vi "5.8G_Range Profile_audiojack_FMCW_demo_exe.vi"() -> ()   [LabVIEW 2015]
doc: "This example demonstrates how to use the Short-time Fourier Transform (STFT Spectrograms) VI to analyze the Time-Frequency spectrogram."
uses:
  <vilib>/Analysis/baseanly.llb/Unit Vector (DBL).vi
  <vilib>/Analysis/baseanly.llb/Mean (DBL).vi
  <vilib>/Analysis/2dsp.llb/Real FFT.vi
  <vilib>/Analysis/2dsp.llb/Complex FFT.vi
  <vilib>/Analysis/0measdsp.llb/Scaled Time Domain Window (DBL).vi
  <vilib>/sound2/lvsound2.llb/Sound Input Read (DBL).vi
  <vilib>/Analysis/NI_AALPro.lvlib
  <vilib>/Analysis/NI_AALBase.lvlib
panel:
  in  "begin offsets":i32=10
  in  "end offsets":i32=200
  in  "window":u32(ring)=1 items=["Rectangle"=0, "Hanning"=1, "Hamming"=2, "Blackman-Harris"=3, "Exact Blackman"=4, "Blackman"=5, "Flat Top"=6, "4 Term B-Harris "=7, "7 Term B-Harris"=8, "Low Sidelobe"=9, "Blackman Nuttall"=11, "Triangle"=30, "Bartlett-Hanning"=31, "Bohman"=32, "Parzen"=33, "Welch"=34, "Kaiser"=60, "Dolph-Chebyshev"=61, "Gaussian"=62]
  in  "ISAR intensify:Minimum":dbl=-30.0
  in  "ISAR intensify: Maximum":dbl
  in  "map selector ISAR":T1(ring)=enum."rainbow"
  out "ISAR":dbl[][](graph)
  in  "range":dbl(slide)=8.722182340272793 min=0.0 max=128.57142857142858 scale=0.0..128.57142857142858
  out "max range":dbl
  out "range resolution":dbl
  out "chirp rate":dbl
  in  "Range intensify:Minimum":dbl=-40.0
  in  "Range intensify:Maximum":dbl
  out "real time chirp frequency":dbl
  in  "FFT length":i32=4096
  in  "chirp frequency":dbl=280.0
  out "Range profile":dbl[][](graph)
  out "average samples per chirp":i32
  in  "threshold":dbl=0.6 format="%0.2f"
  in  "bits per sample":i32=16
  in  "number of channels":i32=2
  in  "sample rate (S/s)":dbl=192000.0
  in  "data length\n(10 x number of samples/ch)":i32=400000 min=10000 max=1000000
  in  "map selector Range profile":T1(ring)=enum."rainbow"
  in  "number of samples/ch":i32=40000 min=1024 max=100000
  in  "Numeric Control":dbl=1.0
  in  "device ID":u32
  in  "Stop":bool
  # "FMCW Radar Realtime Range Detection and ISAR Video"
  # "Version: 4\nZhengyu Peng\nC. Li Lab\nTexas Tech University\nOct. 2016"
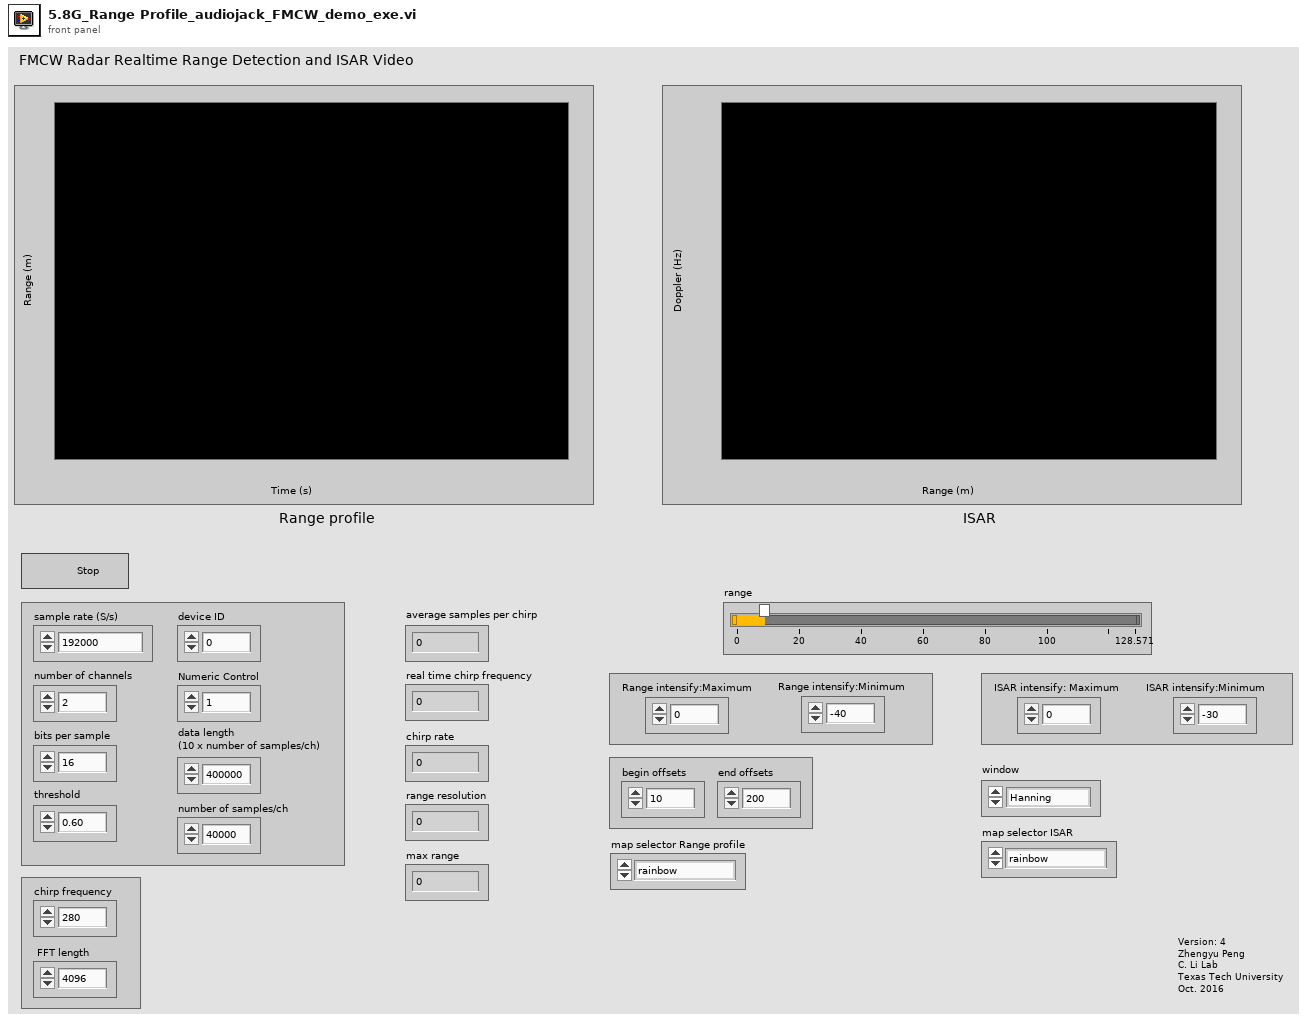
[diagram p1: front panel]
types:
  T1 = enum16{"fire", "rainbow", "grey", "inverse grey", "ice", "original"}
  T2 = cluster{"sample rate (S/s)":dbl, "number of channels":i32, "bits per sample ":i32}
  T3 = typedef "Sound Input Task ID.ctl" = u32
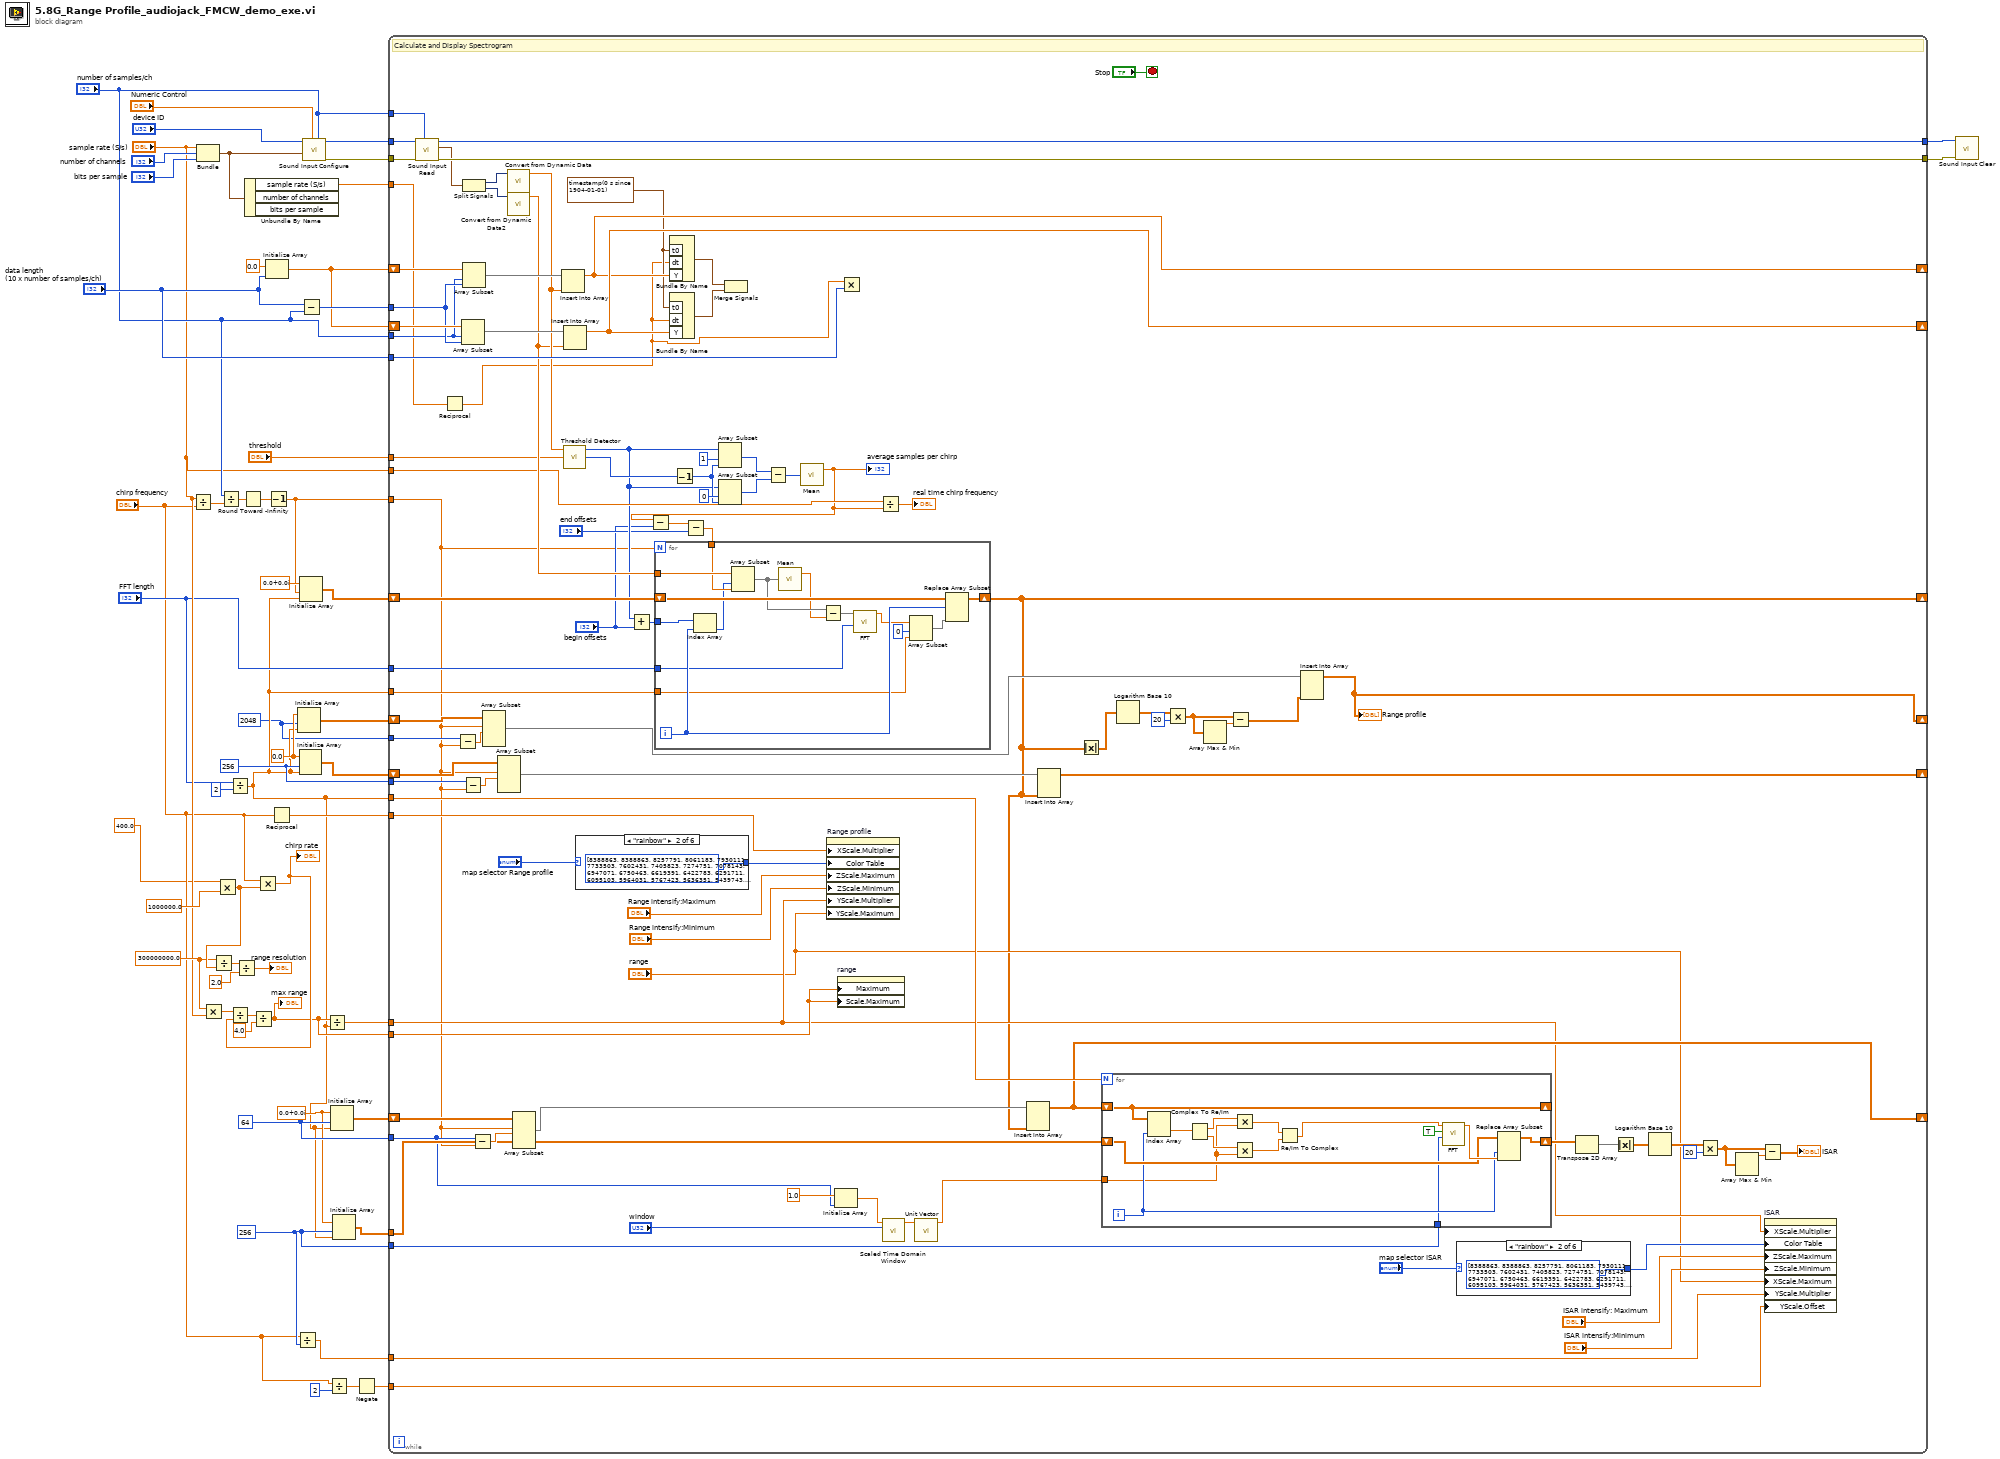
[diagram p0: block diagram]
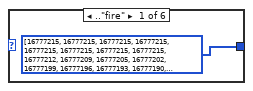
[diagram p2: hidden frame]
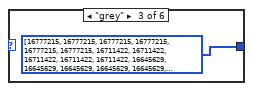
[diagram p3: hidden frame]
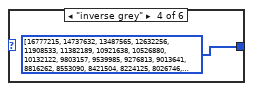
[diagram p4: hidden frame]
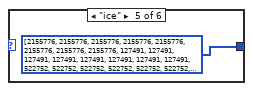
[diagram p5: hidden frame]
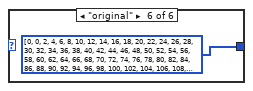
[diagram p6: hidden frame]
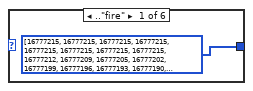
[diagram p7: hidden frame]
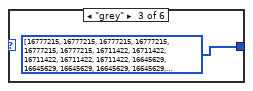
[diagram p8: hidden frame]
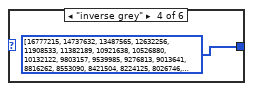
[diagram p9: hidden frame]
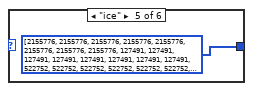
[diagram p10: hidden frame]
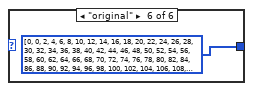
[diagram p11: hidden frame]
diagram:
  w1 = 2048 ("dimension size")
  w7 = 256 ("dimension size")
  w14 = 64 ("dimension size")
  w13 = cdb 0.0+0.0i ("element")
  w25 = 300000000.0 ("x")
  w32 = 256 ("dimension size")
  w4 = 0.0 ("element")
  n1 = Divide(x="sample rate (S/s)", y="chirp frequency") -> (x/y=w36:dbl)
  n2 = Bundle("sample rate (S/s)"="sample rate (S/s)", "number of channels"="number of channels", "bits per sample"="bits per sample") -> (w43:T2)  [unwired: 1 in]
  n3 = Multiply(x=w25, y="sample rate (S/s)") -> (x*y=w24:dbl)
  n4 = Multiply(x=400.0, y=1000000.0) -> (x*y=w29:dbl)
  n5 = Divide(x=w25, y=w29) -> (x/y=w28:dbl)
  n6 = Divide(x="number of samples/ch", y=w36) -> (x/y=w35:dbl)
  n7 = Divide(x="FFT length", y=2) -> (x/y=w3:dbl)
  n8 = Divide(x=w28, y=2.0) -> (x/y=→"range resolution":dbl)
  n9 = Round Toward -Infinity(1:w35) -> (0:w34:dbl)
  n10 = Unbundle By Name(w43) -> ("sample rate (S/s)"=w46:dbl)  [unwired: 2 out]
  n11 = Multiply(x="chirp frequency", y=w29) -> (x*y=w23:dbl)
  "chirp rate" <- w23
  n12 = Divide(x=w24, y=w23) -> (x/y=w22:dbl)
  n13 = Divide(x=w22, y=4.0) -> (x/y=w16:dbl)
  "max range" <- w16
  n14 = Initialize Array(0.0 ("element"), "data length\n(10 x number of samples/ch)") -> (w47:dbl[])
  n15 = Decrement(x=w34) -> (x-1=w33:dbl)
  n16 = Reciprocal(x="chirp frequency") -> (1/x=w31:dbl)
  n17 = Divide(x="chirp frequency", y=w7) -> (x/y=w8:dbl)
  n18 = Initialize Array(w4, w1, w3) -> (w2:dbl[][])
  n19 = Initialize Array(w4, w32, w3) -> (w41:dbl[][])
  n20 = Subtract(x="data length\n(10 x number of samples/ch)", y="number of samples/ch") -> (x-y=w48:i32)
  n21 = Initialize Array(cdb 0.0+0.0i ("element"), w33, w3) -> (w39:cdb[][])
  n22 = call <vilib>:"Sound Input Configure.vi"("number of samples/ch"="number of samples/ch", "sample mode"="Numeric Control", "sound format"=w43, "device ID"="device ID") -> ("error out"=w52:errorcluster, "task ID"=w54:T3)  [unwired: 6 in]
  n23 = Divide(x=w16, y=w3) -> (x/y=w17:dbl)
  n24 = Divide(x="chirp frequency", y=2) -> (x/y=w10:dbl)
  n25 = Initialize Array(w13, w14, w3) -> (w15:cdb[][])
  n26 = Initialize Array(w13, w7, w3) -> (w12:cdb[][])
  n27 = Negate(x=w10) -> (-x=w9:dbl)
  n28 = while {
    tunnel: w54 -> [w152]
    tunnel: "number of samples/ch" -> [w151]
    tunnel: w52 -> [w150]
    tunnel: [w149] -> w51
    tunnel: [w148] -> w50
    shift-right: [w132] -> _
    shift-left: w47 -> [w144]
    tunnel: w48 -> [w141]
    shift-right: [w134] -> _
    shift-left: w47 -> [w142]
    tunnel: "number of samples/ch" -> [w137]
    tunnel: w46 -> [w133]
    tunnel: "data length\n(10 x number of samples/ch)" -> [w135]
    shift-right: [w60] -> _
    shift-left: w41 -> [w123]
    shift-right: [w57] -> _
    shift-left: w39 -> [w122]
    tunnel: "threshold" -> [w113]
    tunnel: w33 -> [w62]
    tunnel: "sample rate (S/s)" -> [w112]
    tunnel: "FFT length" -> [w110]
    tunnel: w32 -> [w109]
    tunnel: w31 -> [w66]
    tunnel: w17 -> [w83]
    tunnel: w3 -> [w104]
    tunnel: w16 -> [w103]
    shift-right: [w98] -> _
    shift-left: w15 -> [w102]
    tunnel: w14 -> [w86]
    tunnel: w3 -> [w99]
    tunnel: w12 -> [w97]
    tunnel: w7 -> [w76]
    tunnel: w9 -> [w74]
    tunnel: w8 -> [w75]
    shift-right: [w56] -> _
    shift-left: w2 -> [w65]
    tunnel: w1 -> [w64]
    stop <- "Stop" stop-if-true
    w120 = timestamp(0 s since 1904-01-01) ("t0")
    # "Calculate and Display Spectrogram"
    n29 = call-poly <vilib>:"Sound Input Read.vi"("number of samples/ch"=w151, "error in (no error)"=w150, "task ID"=w152) -> ("error out"=w148:errorcluster, "data"=w145:waveform(dbl)[], "task ID out"=w149:T3)  [unwired: 6 in]
    n30 = Reciprocal(x=w133) -> (1/x=w119:dbl)
    n31 = Subtract(x=w64, y=w62) -> (x-y=w63:dbl)
    n32 = Array Subset(array=w142, index=w137, length=w141) -> (w140:dbl[])
    n33 = Subtract(x=w109, y=w62) -> (x-y=w108:dbl)
    n34 = Split Signals(w145) -> (w147:dynamicdata, w146:dynamicdata)  [unwired: 2 out]
    n35 = Array Subset(array=w144, index=w137, length=w141) -> (w143:dbl[])
    n36 = Subtract(x=w86, y=w62) -> (x-y=w101:dbl)
    n37 = Array Subset(array=w65, index (row)=w62, length (row)=w63) -> (w59:dbl[][])  [unwired: 2 in]
    n38 = Array Subset(array=w123, index (row)=w62, length (row)=w108) -> (w118:dbl[][])  [unwired: 2 in]
    n39 = call "Convert from Dynamic Data"("Dynamic Data Type"=w147) -> ("Array"=w131:dbl[])  [unwired: 3 out]
    n40 = call "Convert from Dynamic Data2"("Dynamic Data Type"=w146) -> ("Array"=w121:dbl[])  [unwired: 3 out]
    n41 = Array Subset(array=w102, index (row)=w62, length (row)=w101) -> (w100:cdb[][])  [unwired: 2 in]
    n42 = Insert Into Array(array=w143, new element=w131) -> (w132:dbl[])  [unwired: 1 in]
    n43 = call <vilib>:"Threshold Detector.vi"("threshold"=w113, "X"=w131) -> ("count"=w126:i32, "Indices"=w73:i32[])  [unwired: 1 in, 1 out]
    n44 = Insert Into Array(array=w140, new element=w121) -> (w134:dbl[])  [unwired: 1 in]
    n45 = case shown="\"rainbow\"" "map selector Range profile" {
      tunnel: [u32[] [16777215, 16777215, 16777215, 16777215, 16777215, 16777215, 16777215, 16777215, 16777212, 16777209, 16777205, 16777202, 16777199, 16777196, 16777193, 16777190, 16777186, 16777183, 16777180, 16777177, 16777174, 16777170, 16777167, 16777164, 16777161, 16777158, 16777154, 16777151, 16777148, 16777145, 16777142, 16777139, 16777135, 16777132, 16777129, 16777126, 16777123, 16777119, 16777116, 16777113, 16777110, 16777107, 16777103, 16777100, 16777097, 16777094, 16777091, 16777088, 16777084, 16777081, 16777078, 16777075, 16777072, 16777068, 16777065, 16777062, 16777059, 16777056, 16777052, 16777049, 16777046, 16777043, 16777040, 16777037, 16777033, 16777030, 16777027, 16777024, 16777021, 16777017, 16777014, 16777011, 16777008, 16777005, 16777001, 16776998, 16776995, 16776992, 16776989, 16776986, 16776982, 16776979, 16776976, 16776973, 16776970, 16776966, 16776963, 16776960, 16776192, 16775424, 16774400, 16773632, 16772864, 16772096, 16771328, 16770560, 16769536, 16768768, 16768000, 16767232, 16766464, 16765440, 16764672, 16763904, 16763136, 16762368, 16761344, 16760576, 16759808, 16759040, 16758272, 16757504, 16756480, 16755712, 16754944, 16754176, 16753408, 16752384, 16751616, 16750848, 16750080, 16749312, 16748288, 16747520, 16746752, 16745984, 16745216, 16744448, 16743424, 16742656, 16741888, 16741120, 16740352, 16739328, 16738560, 16737792, 16737024, 16736256, 16735232, 16734464, 16733696, 16732928, 16732160, 16731392, 16730368, 16729600, 16728832, 16728064, 16727296, 16726272, 16725504, 16724736, 16723968, 16723200, 16722176, 16721408, 16720640, 16719872, 16719104, 16718336, 16717312, 16716544, 16715776, 16715008, 16714240, 16713216, 16712448, 16711680, 16515072, 16318464, 16056320, 15859712, 15663104, 15466496, 15269888, 15073280, 14811136, 14614528, 14417920, 14221312, 14024704, 13762560, 13565952, 13369344, 13172736, 12976128, 12713984, 12517376, 12320768, 12124160, 11927552, 11730944, 11468800, 11272192, 11075584, 10878976, 10682368, 10420224, 10223616, 10027008, 9830400, 9633792, 9371648, 9175040, 8978432, 8781824, 8585216, 8388608, 8126464, 7929856, 7733248, 7536640, 7340032, 7077888, 6881280, 6684672, 6488064, 6291456, 6029312, 5832704, 5636096, 5439488, 5242880, 5046272, 4784128, 4587520, 4390912, 4194304, 3997696, 3735552, 3538944, 3342336, 3145728, 2949120, 2686976, 2490368, 2293760, 2097152, 1900544, 1703936, 1441792, 1245184, 1048576, 851968, 655360, 393216, 196608, 65793, 65793, 65793, 65793, 65793, 65793, 65793, 65793, 0] ("256 fire") u32[] [8388863, 8388863, 8257791, 8061183, 7930111, 7733503, 7602431, 7405823, 7274751, 7078143, 6947071, 6750463, 6619391, 6422783, 6291711, 6095103, 5964031, 5767423, 5636351, 5439743, 5308671, 5112063, 4980991, 4784383, 4653311, 4456703, 4325631, 4129023, 3932415, 3801343, 3604735, 3473663, 3277055, 3145983, 2949375, 2818303, 2621695, 2490623, 2294015, 2162943, 1966335, 1835263, 1638655, 1507583, 1310975, 1179903, 983295, 852223, 655615, 524543, 327935, 196863, 511, 1791, 3071, 4351, 5631, 6911, 8191, 9471, 10751, 12031, 13311, 14591, 15871, 17151, 18431, 19711, 20991, 22271, 23551, 24831, 26111, 27391, 28671, 29951, 31231, 32511, 33791, 35071, 36351, 37631, 38911, 40191, 41471, 42751, 44031, 45311, 46591, 47871, 49151, 50431, 51711, 52991, 54271, 55551, 56831, 58111, 59391, 60671, 61951, 63231, 64511, 65532, 65527, 65522, 65517, 65512, 65507, 65502, 65497, 65492, 65487, 65482, 65477, 65472, 65467, 65462, 65457, 65452, 65447, 65442, 65437, 65432, 65427, 65422, 65417, 65412, 65407, 65402, 65397, 65392, 65387, 65382, 65377, 65372, 65367, 65362, 65357, 65352, 65347, 65342, 65337, 65332, 65327, 65322, 65317, 65312, 65307, 65302, 65297, 65292, 65287, 65282, 261888, 589568, 917248, 1244928, 1572608, 1900288, 2227968, 2555648, 2883328, 3211008, 3538688, 3866368, 4194048, 4521728, 4849408, 5177088, 5504768, 5832448, 6160128, 6487808, 6815488, 7143168, 7470848, 7798528, 8126208, 8453888, 8781568, 9109248, 9436928, 9764608, 10092288, 10419968, 10747648, 11075328, 11403008, 11730688, 12058368, 12386048, 12713728, 13041408, 13369088, 13696768, 14024448, 14352128, 14679808, 15007488, 15335168, 15662848, 15990528, 16318208, 16645888, 16775936, 16774656, 16773376, 16772096, 16770816, 16769536, 16768256, 16766976, 16765696, 16764416, 16763136, 16761856, 16760576, 16759296, 16758016, 16756736, 16755456, 16754176, 16752896, 16751616, 16750336, 16749056, 16747776, 16746496, 16745216, 16743936, 16742656, 16741376, 16740096, 16738816, 16737536, 16736256, 16734976, 16733696, 16732416, 16731136, 16729856, 16728576, 16727296, 16726016, 16724736, 16723456, 16722176, 16720896, 16719616, 16718336, 16717056, 16715776, 16714496, 16713216, 16711680] ("rainbow") u32[] [16777215, 16777215, 16777215, 16777215, 16777215, 16777215, 16711422, 16711422, 16711422, 16711422, 16711422, 16645629, 16645629, 16645629, 16645629, 16645629, 16645629, 16579836, 16579836, 16579836, 16579836, 16579836, 16514043, 16514043, 16514043, 16514043, 16514043, 16448250, 16448250, 16448250, 16448250, 16448250, 16316664, 16382457, 16382457, 16382457, 16382457, 16316664, 16316664, 16316664, 16316664, 16250871, 16250871, 16250871, 16250871, 16250871, 16185078, 16185078, 16185078, 16185078, 16119285, 16119285, 16119285, 16119285, 16119285, 16053492, 16053492, 16053492, 16053492, 15987699, 15987699, 15987699, 15987699, 15921906, 15987699, 15921906, 15921906, 15856113, 15856113, 15856113, 15856113, 15856113, 15790320, 15790320, 15790320, 15724527, 15724527, 15724527, 15724527, 15658734, 15658734, 15658734, 15658734, 15592941, 15592941, 15592941, 15592941, 15527148, 15527148, 15527148, 15461355, 15461355, 15461355, 15461355, 15395562, 15395562, 15395562, 15395562, 15329769, 15329769, 15329769, 15263976, 15263976, 15263976, 15198183, 15198183, 15198183, 15198183, 15132390, 15132390, 15132390, 15066597, 15066597, 15066597, 15000804, 15000804, 15000804, 14935011, 14935011, 14935011, 14869218, 14869218, 14869218, 14803425, 14803425, 14803425, 14737632, 14737632, 14671839, 14671839, 14671839, 14606046, 14606046, 14606046, 14540253, 14540253, 14540253, 14474460, 14474460, 14408667, 14408667, 14408667, 14342874, 14342874, 14277081, 14277081, 14277081, 14211288, 14211288, 14145495, 14145495, 14079702, 14079702, 14013909, 14013909, 14013909, 13948116, 13948116, 13882323, 13882323, 13816530, 13816530, 13750737, 13750737, 13684944, 13684944, 13619151, 13619151, 13553358, 13553358, 13487565, 13487565, 13421772, 13421772, 13355979, 13290186, 13290186, 13224393, 13224393, 13158600, 13092807, 13092807, 13027014, 13027014, 12961221, 12895428, 12895428, 12829635, 12763842, 12763842, 12698049, 12632256, 12566463, 12566463, 12500670, 12434877, 12434877, 12369084, 12303291, 12237498, 12171705, 12171705, 12105912, 12040119, 11974326, 11908533, 11842740, 11776947, 11711154, 11645361, 11579568, 11513775, 11447982, 11382189, 11316396, 11250603, 11184810, 11119017, 10987431, 10921638, 10855845, 10790052, 10658466, 10592673, 10461087, 10395294, 10329501, 10197915, 10066329, 10000536, 9868950, 9737364, 9605778, 9474192, 9342606, 9211020, 9079434, 8882055, 8750469, 8553090, 8421504, 8224125, 7960953, 7763574, 7500402, 7237230, 6974058, 6645093, 6316128, 5855577, 5395026, 4868682, 4210752, 3289650, 2105376, 0] ("256 log up") u32[] [16777215, 14737632, 13487565, 12632256, 11908533, 11382189, 10921638, 10526880, 10132122, 9803157, 9539985, 9276813, 9013641, 8816262, 8553090, 8421504, 8224125, 8026746, 7895160, 7697781, 7566195, 7434609, 7303023, 7171437, 7039851, 6908265, 6776679, 6710886, 6579300, 6447714, 6381921, 6316128, 6184542, 6118749, 5987163, 5921370, 5855577, 5789784, 5658198, 5592405, 5526612, 5460819, 5395026, 5329233, 5263440, 5197647, 5131854, 5066061, 5000268, 4934475, 4868682, 4802889, 4737096, 4671303, 4605510, 4605510, 4539717, 4473924, 4408131, 4342338, 4342338, 4276545, 4210752, 4210752, 4144959, 4079166, 4013373, 4013373, 3947580, 3881787, 3881787, 3815994, 3750201, 3750201, 3684408, 3684408, 3618615, 3552822, 3552822, 3487029, 3487029, 3421236, 3421236, 3355443, 3289650, 3289650, 3223857, 3223857, 3158064, 3158064, 3092271, 3092271, 3026478, 3026478, 2960685, 2960685, 2894892, 2894892, 2829099, 2829099, 2763306, 2763306, 2763306, 2697513, 2697513, 2631720, 2631720, 2565927, 2565927, 2500134, 2500134, 2500134, 2434341, 2434341, 2368548, 2368548, 2368548, 2302755, 2302755, 2236962, 2236962, 2236962, 2171169, 2171169, 2171169, 2105376, 2105376, 2105376, 2039583, 2039583, 1973790, 1973790, 1973790, 1907997, 1907997, 1907997, 1842204, 1842204, 1842204, 1776411, 1776411, 1776411, 1710618, 1710618, 1710618, 1644825, 1644825, 1644825, 1579032, 1579032, 1579032, 1579032, 1513239, 1513239, 1513239, 1447446, 1447446, 1447446, 1381653, 1381653, 1381653, 1381653, 1315860, 1315860, 1315860, 1315860, 1250067, 1250067, 1250067, 1184274, 1184274, 1184274, 1184274, 1118481, 1118481, 1118481, 1118481, 1052688, 1052688, 1052688, 1052688, 986895, 986895, 986895, 921102, 921102, 921102, 921102, 921102, 855309, 855309, 855309, 855309, 789516, 789516, 789516, 789516, 723723, 723723, 723723, 723723, 657930, 657930, 657930, 657930, 657930, 592137, 592137, 592137, 592137, 526344, 526344, 526344, 526344, 526344, 460551, 460551, 460551, 460551, 460551, 394758, 394758, 394758, 394758, 328965, 328965, 328965, 328965, 328965, 263172, 263172, 263172, 263172, 263172, 197379, 197379, 197379, 197379, 197379, 131586, 131586, 131586, 131586, 131586, 131586, 65793, 65793, 65793, 65793, 65793, 0, 0, 0, 0, 0, 0] ("256 log down") u32[] [2155776, 2155776, 2155776, 2155776, 2155776, 2155776, 2155776, 2155776, 127491, 127491, 127491, 127491, 127491, 127491, 127491, 127491, 522752, 522752, 522752, 522752, 522752, 522752, 522752, 522752, 64018, 64018, 64018, 64018, 64018, 64018, 64018, 64018, 63778, 63778, 63778, 63778, 63778, 63778, 63778, 63778, 63790, 63790, 63790, 63790, 63790, 63790, 63790, 63790, 63797, 63797, 63797, 63797, 63797, 63797, 63797, 63797, 63807, 63807, 63807, 63807, 63807, 63807, 63807, 63807, 64068, 64068, 64068, 64068, 64068, 64068, 64068, 64068, 63828, 63828, 63828, 63828, 63828, 63828, 63828, 63828, 63833, 63833, 63833, 63833, 63833, 63833, 63833, 63833, 63836, 63836, 63836, 63836, 63836, 63836, 63836, 63836, 63836, 63836, 63836, 63836, 63836, 63836, 63836, 63836, 61790, 61790, 61790, 61790, 61790, 61790, 61790, 61790, 58464, 58464, 58464, 58464, 58464, 58464, 58464, 58464, 55387, 55387, 55387, 55387, 55387, 55387, 55387, 55387, 51286, 51286, 51286, 51286, 51286, 51286, 51286, 51286, 47440, 47440, 47440, 47440, 47440, 47440, 47440, 47440, 40284, 40284, 40284, 40284, 40284, 40284, 40284, 40284, 34154, 34154, 34154, 34154, 34154, 34154, 34154, 34154, 28540, 28540, 28540, 28540, 28540, 28540, 28540, 28540, 20113, 20113, 20113, 20113, 20113, 20113, 20113, 20113, 12193, 12193, 12193, 12193, 12193, 12193, 12193, 12193, 12714, 12714, 12714, 12714, 12714, 12714, 12714, 12714, 7351, 7351, 7351, 7351, 7351, 7351, 7351, 7351, 4800, 4800, 4800, 4800, 4800, 4800, 4800, 4800, 195, 195, 195, 195, 195, 195, 195, 195, 189, 189, 189, 189, 189, 189, 189, 189, 183, 183, 183, 183, 183, 183, 183, 183, 175, 175, 175, 175, 175, 175, 175, 175, 164, 164, 164, 164, 164, 164, 164, 164, 155, 155, 155, 155, 155, 155, 155, 155] ("32 ice") u32[] [0, 0, 2, 4, 6, 8, 10, 12, 14, 16, 18, 20, 22, 24, 26, 28, 30, 32, 34, 36, 38, 40, 42, 44, 46, 48, 50, 52, 54, 56, 58, 60, 62, 64, 66, 68, 70, 72, 74, 76, 78, 80, 82, 84, 86, 88, 90, 92, 94, 96, 98, 100, 102, 104, 106, 108, 110, 112, 114, 116, 118, 120, 122, 124, 126, 128, 130, 132, 134, 136, 138, 140, 142, 144, 146, 148, 150, 152, 154, 156, 158, 160, 162, 164, 166, 168, 170, 172, 174, 176, 178, 180, 182, 184, 186, 188, 190, 192, 194, 196, 198, 200, 202, 204, 206, 208, 210, 212, 214, 216, 218, 220, 222, 224, 226, 228, 230, 232, 234, 236, 238, 240, 242, 244, 246, 248, 250, 252, 255, 131839, 263423, 395007, 526591, 658175, 789759, 921343, 1052927, 1184511, 1316095, 1447679, 1579263, 1710847, 1842431, 1974015, 2105599, 2237183, 2368767, 2500351, 2631935, 2763519, 2895103, 3026687, 3158271, 3289855, 3421439, 3553023, 3684607, 3816191, 3947775, 4079359, 4210943, 4342527, 4474111, 4605695, 4737279, 4868863, 5000447, 5132031, 5263615, 5395199, 5526783, 5658367, 5789951, 5921535, 6053119, 6184703, 6316287, 6447871, 6579455, 6711039, 6842623, 6974207, 7105791, 7237375, 7368959, 7500543, 7632127, 7763711, 7895295, 8026879, 8158463, 8290047, 8421631, 8553215, 8684799, 8816383, 8947967, 9079551, 9211135, 9342719, 9474303, 9605887, 9737471, 9869055, 10000639, 10132223, 10263807, 10395391, 10526975, 10658559, 10790143, 10921727, 11053311, 11184895, 11316479, 11448063, 11579647, 11711231, 11842815, 11974399, 12105983, 12237567, 12369151, 12500735, 12632319, 12763903, 12895487, 13027071, 13158655, 13290239, 13421823, 13553407, 13684991, 13816575, 13948159, 14079743, 14211327, 14342911, 14474495, 14606079, 14737663, 14869247, 15000831, 15132415, 15263999, 15395583, 15527167, 15658751, 15790335, 15921919, 16053503, 16185087, 16316671, 16448255, 16579839, 16777215] ("original")] -> w107
      frame .."fire" {
      }
      frame "rainbow" {
      }
      frame "grey" {
      }
      frame "inverse grey" {
      }
      frame "ice" {
      }
      frame "original" {
      }
    }
    n46 = Add(x=w73, y="begin offsets") -> (x+y=w72:i32[])
    n47 = Bundle By Name("t0"=w120, "dt"=w119, "Y"=w132) -> (w139:waveform(dbl))  [unwired: 1 out]
    n48 = Bundle By Name("t0"=w120, "dt"=w119, "Y"=w134) -> (w136:waveform(dbl))  [unwired: 1 out]
    n49 = Decrement(x=w126) -> (x-1=w125:i32)
    n50 = Array Subset(array=w73, index=1, length=w125) -> (w128:i32[])
    n51 = Array Subset(array=w73, index=0, length=w125) -> (w127:i32[])
    n52 = Merge Signals(w139, w136) -> ()  [unwired: 1 out]
    n53 = Subtract(x=w128, y=w127) -> (x-y=w124:i32[])
    n54 = call-poly <vilib>:"Mean.vi"("X"=w124) -> ("mean"=w69:dbl)  [unwired: 1 out]
    "average samples per chirp" <- w69
    n55 = Subtract(x=w69, y="begin offsets") -> (x-y=w67:dbl)
    n56 = Subtract(x=w67, y="end offsets") -> (x-y=w71:dbl)
    n57 = for {
      N: w62 -> [_]
      tunnel: w121 -> [w187]
      tunnel: w71 -> [w186]
      tunnel: w72 -> [w185]
      shift-right: [w183] -> w57
      shift-left: w122 -> [w188]
      tunnel: w110 -> [w181]
      tunnel: w104 -> [w174]
      i -> [w182]
      n58 = Index Array(array=w185, index=w182) -> (element=w184:i32)
      n59 = Array Subset(array=w187, index=w184, length=w186) -> (w180:dbl[])
      n60 = call-poly <vilib>:"Mean.vi"("X"=w180) -> ("mean"=w179:dbl)  [unwired: 1 out]
      n61 = Subtract(x=w180, y=w179) -> (x-y=w178:dbl[])
      n62 = call-poly <vilib>:"FFT.vi"("FFT size"=w181, "X"=w178) -> ("FFT {X}"=w177:cdb[])  [unwired: 8 in, 1 out]
      n63 = Array Subset(array=w177, index=0, length=w174) -> (w176:cdb[])
      n64 = Replace Array Subset(array=w188, new element=w176, index (row)=w182) -> (w183:cdb[][])  [unwired: 1 in]
    }
    n65 = property on="Range profile" class="IntGraph (strict)"("XScale.Multiplier"=w66, "Color Table"=w107, "ZScale.Maximum"="Range intensify:Maximum", "ZScale.Minimum"="Range intensify:Minimum", "YScale.Multiplier"=w83, "YScale.Maximum"="range") -> ()  [unwired: 2 in, 2 out]
    n66 = Initialize Array(1.0 ("element"), w86) -> (w85:dbl[])
    n67 = property on="range" class="Slide (strict)"("Maximum"=w103, "Scale.Maximum"=w103) -> ()  [unwired: 2 in, 2 out]
    n68 = Multiply(x=w119, y=w135) -> ()  [unwired: 1 out]
    n69 = Divide(x=w112, y=w69) -> (x/y=→"real time chirp frequency":dbl)
    n70 = call-poly <vilib>:"Scaled Time Domain Window.vi"("window"="window", "X"=w85) -> ("Windowed X"=w88:dbl[])  [unwired: 7 in, 2 out]
    n71 = call-poly <vilib>:"Unit Vector.vi"("Input Vector"=w88) -> ("Unit Vector"=w84:dbl[])  [unwired: 8 in, 2 out]
    n72 = Insert Into Array(array=w100, new element=w57) -> (w98:cdb[][])  [unwired: 2 in]
    n73 = Insert Into Array(array=w118, new element=w57) -> (w60:dbl[][])  [unwired: 2 in]
    n74 = Absolute Value(x=w57) -> (abs(x)=w61:dbl[][])
    n75 = for {
      N: w99 -> [_]
      shift-right: [w168] -> w90
      shift-left: w97 -> [w171]
      shift-right: [w170] -> _
      shift-left: w98 -> [w170]
      tunnel: w84 -> [w164]
      tunnel: w76 -> [w160]
      i -> [w169]
      n76 = Index Array(array=w170, index (col)=w169) -> (element=w167:cdb[])  [unwired: 1 in]
      n77 = Complex To Re/Im(x + iy=w167) -> (x=w166:dbl[], y=w165:dbl[])
      n78 = Multiply(x=w166, y=w164) -> (x*y=w163:dbl[])
      n79 = Multiply(x=w165, y=w164) -> (x*y=w162:dbl[])
      n80 = Re/Im To Complex(1:w162, 2:w163) -> (0:w161:cdb[])
      n81 = call-poly <vilib>:"FFT.vi"("FFT size"=w160, "shift?"=TRUE, "X"=w161) -> ("FFT {X}"=w172:cdb[])  [unwired: 7 in, 1 out]
      n82 = Replace Array Subset(array=w171, new element=w172, index (col)=w169) -> (w168:cdb[][])  [unwired: 1 in]
    }
    n83 = Logarithm Base 10(1:w61) -> (0:w114:dbl[][])
    n84 = Multiply(x=w114, y=i8 20 ("t")) -> (x*y=w116:dbl[][])
    n85 = Array Max & Min(array=w116) -> (max value=w117:dbl)  [unwired: 3 out]
    n86 = Subtract(x=w116, y=w117) -> (x-y=w58:dbl[][])
    n87 = Insert Into Array(array=w59, new element=w58) -> (w56:dbl[][])  [unwired: 2 in]
    "Range profile" <- w56
    n88 = case shown="\"rainbow\"" "map selector ISAR" {
      tunnel: [u32[] [16777215, 16777215, 16777215, 16777215, 16777215, 16777215, 16777215, 16777215, 16777212, 16777209, 16777205, 16777202, 16777199, 16777196, 16777193, 16777190, 16777186, 16777183, 16777180, 16777177, 16777174, 16777170, 16777167, 16777164, 16777161, 16777158, 16777154, 16777151, 16777148, 16777145, 16777142, 16777139, 16777135, 16777132, 16777129, 16777126, 16777123, 16777119, 16777116, 16777113, 16777110, 16777107, 16777103, 16777100, 16777097, 16777094, 16777091, 16777088, 16777084, 16777081, 16777078, 16777075, 16777072, 16777068, 16777065, 16777062, 16777059, 16777056, 16777052, 16777049, 16777046, 16777043, 16777040, 16777037, 16777033, 16777030, 16777027, 16777024, 16777021, 16777017, 16777014, 16777011, 16777008, 16777005, 16777001, 16776998, 16776995, 16776992, 16776989, 16776986, 16776982, 16776979, 16776976, 16776973, 16776970, 16776966, 16776963, 16776960, 16776192, 16775424, 16774400, 16773632, 16772864, 16772096, 16771328, 16770560, 16769536, 16768768, 16768000, 16767232, 16766464, 16765440, 16764672, 16763904, 16763136, 16762368, 16761344, 16760576, 16759808, 16759040, 16758272, 16757504, 16756480, 16755712, 16754944, 16754176, 16753408, 16752384, 16751616, 16750848, 16750080, 16749312, 16748288, 16747520, 16746752, 16745984, 16745216, 16744448, 16743424, 16742656, 16741888, 16741120, 16740352, 16739328, 16738560, 16737792, 16737024, 16736256, 16735232, 16734464, 16733696, 16732928, 16732160, 16731392, 16730368, 16729600, 16728832, 16728064, 16727296, 16726272, 16725504, 16724736, 16723968, 16723200, 16722176, 16721408, 16720640, 16719872, 16719104, 16718336, 16717312, 16716544, 16715776, 16715008, 16714240, 16713216, 16712448, 16711680, 16515072, 16318464, 16056320, 15859712, 15663104, 15466496, 15269888, 15073280, 14811136, 14614528, 14417920, 14221312, 14024704, 13762560, 13565952, 13369344, 13172736, 12976128, 12713984, 12517376, 12320768, 12124160, 11927552, 11730944, 11468800, 11272192, 11075584, 10878976, 10682368, 10420224, 10223616, 10027008, 9830400, 9633792, 9371648, 9175040, 8978432, 8781824, 8585216, 8388608, 8126464, 7929856, 7733248, 7536640, 7340032, 7077888, 6881280, 6684672, 6488064, 6291456, 6029312, 5832704, 5636096, 5439488, 5242880, 5046272, 4784128, 4587520, 4390912, 4194304, 3997696, 3735552, 3538944, 3342336, 3145728, 2949120, 2686976, 2490368, 2293760, 2097152, 1900544, 1703936, 1441792, 1245184, 1048576, 851968, 655360, 393216, 196608, 65793, 65793, 65793, 65793, 65793, 65793, 65793, 65793, 0] ("256 fire") u32[] [8388863, 8388863, 8257791, 8061183, 7930111, 7733503, 7602431, 7405823, 7274751, 7078143, 6947071, 6750463, 6619391, 6422783, 6291711, 6095103, 5964031, 5767423, 5636351, 5439743, 5308671, 5112063, 4980991, 4784383, 4653311, 4456703, 4325631, 4129023, 3932415, 3801343, 3604735, 3473663, 3277055, 3145983, 2949375, 2818303, 2621695, 2490623, 2294015, 2162943, 1966335, 1835263, 1638655, 1507583, 1310975, 1179903, 983295, 852223, 655615, 524543, 327935, 196863, 511, 1791, 3071, 4351, 5631, 6911, 8191, 9471, 10751, 12031, 13311, 14591, 15871, 17151, 18431, 19711, 20991, 22271, 23551, 24831, 26111, 27391, 28671, 29951, 31231, 32511, 33791, 35071, 36351, 37631, 38911, 40191, 41471, 42751, 44031, 45311, 46591, 47871, 49151, 50431, 51711, 52991, 54271, 55551, 56831, 58111, 59391, 60671, 61951, 63231, 64511, 65532, 65527, 65522, 65517, 65512, 65507, 65502, 65497, 65492, 65487, 65482, 65477, 65472, 65467, 65462, 65457, 65452, 65447, 65442, 65437, 65432, 65427, 65422, 65417, 65412, 65407, 65402, 65397, 65392, 65387, 65382, 65377, 65372, 65367, 65362, 65357, 65352, 65347, 65342, 65337, 65332, 65327, 65322, 65317, 65312, 65307, 65302, 65297, 65292, 65287, 65282, 261888, 589568, 917248, 1244928, 1572608, 1900288, 2227968, 2555648, 2883328, 3211008, 3538688, 3866368, 4194048, 4521728, 4849408, 5177088, 5504768, 5832448, 6160128, 6487808, 6815488, 7143168, 7470848, 7798528, 8126208, 8453888, 8781568, 9109248, 9436928, 9764608, 10092288, 10419968, 10747648, 11075328, 11403008, 11730688, 12058368, 12386048, 12713728, 13041408, 13369088, 13696768, 14024448, 14352128, 14679808, 15007488, 15335168, 15662848, 15990528, 16318208, 16645888, 16775936, 16774656, 16773376, 16772096, 16770816, 16769536, 16768256, 16766976, 16765696, 16764416, 16763136, 16761856, 16760576, 16759296, 16758016, 16756736, 16755456, 16754176, 16752896, 16751616, 16750336, 16749056, 16747776, 16746496, 16745216, 16743936, 16742656, 16741376, 16740096, 16738816, 16737536, 16736256, 16734976, 16733696, 16732416, 16731136, 16729856, 16728576, 16727296, 16726016, 16724736, 16723456, 16722176, 16720896, 16719616, 16718336, 16717056, 16715776, 16714496, 16713216, 16711680] ("rainbow") u32[] [16777215, 16777215, 16777215, 16777215, 16777215, 16777215, 16711422, 16711422, 16711422, 16711422, 16711422, 16645629, 16645629, 16645629, 16645629, 16645629, 16645629, 16579836, 16579836, 16579836, 16579836, 16579836, 16514043, 16514043, 16514043, 16514043, 16514043, 16448250, 16448250, 16448250, 16448250, 16448250, 16316664, 16382457, 16382457, 16382457, 16382457, 16316664, 16316664, 16316664, 16316664, 16250871, 16250871, 16250871, 16250871, 16250871, 16185078, 16185078, 16185078, 16185078, 16119285, 16119285, 16119285, 16119285, 16119285, 16053492, 16053492, 16053492, 16053492, 15987699, 15987699, 15987699, 15987699, 15921906, 15987699, 15921906, 15921906, 15856113, 15856113, 15856113, 15856113, 15856113, 15790320, 15790320, 15790320, 15724527, 15724527, 15724527, 15724527, 15658734, 15658734, 15658734, 15658734, 15592941, 15592941, 15592941, 15592941, 15527148, 15527148, 15527148, 15461355, 15461355, 15461355, 15461355, 15395562, 15395562, 15395562, 15395562, 15329769, 15329769, 15329769, 15263976, 15263976, 15263976, 15198183, 15198183, 15198183, 15198183, 15132390, 15132390, 15132390, 15066597, 15066597, 15066597, 15000804, 15000804, 15000804, 14935011, 14935011, 14935011, 14869218, 14869218, 14869218, 14803425, 14803425, 14803425, 14737632, 14737632, 14671839, 14671839, 14671839, 14606046, 14606046, 14606046, 14540253, 14540253, 14540253, 14474460, 14474460, 14408667, 14408667, 14408667, 14342874, 14342874, 14277081, 14277081, 14277081, 14211288, 14211288, 14145495, 14145495, 14079702, 14079702, 14013909, 14013909, 14013909, 13948116, 13948116, 13882323, 13882323, 13816530, 13816530, 13750737, 13750737, 13684944, 13684944, 13619151, 13619151, 13553358, 13553358, 13487565, 13487565, 13421772, 13421772, 13355979, 13290186, 13290186, 13224393, 13224393, 13158600, 13092807, 13092807, 13027014, 13027014, 12961221, 12895428, 12895428, 12829635, 12763842, 12763842, 12698049, 12632256, 12566463, 12566463, 12500670, 12434877, 12434877, 12369084, 12303291, 12237498, 12171705, 12171705, 12105912, 12040119, 11974326, 11908533, 11842740, 11776947, 11711154, 11645361, 11579568, 11513775, 11447982, 11382189, 11316396, 11250603, 11184810, 11119017, 10987431, 10921638, 10855845, 10790052, 10658466, 10592673, 10461087, 10395294, 10329501, 10197915, 10066329, 10000536, 9868950, 9737364, 9605778, 9474192, 9342606, 9211020, 9079434, 8882055, 8750469, 8553090, 8421504, 8224125, 7960953, 7763574, 7500402, 7237230, 6974058, 6645093, 6316128, 5855577, 5395026, 4868682, 4210752, 3289650, 2105376, 0] ("256 log up") u32[] [16777215, 14737632, 13487565, 12632256, 11908533, 11382189, 10921638, 10526880, 10132122, 9803157, 9539985, 9276813, 9013641, 8816262, 8553090, 8421504, 8224125, 8026746, 7895160, 7697781, 7566195, 7434609, 7303023, 7171437, 7039851, 6908265, 6776679, 6710886, 6579300, 6447714, 6381921, 6316128, 6184542, 6118749, 5987163, 5921370, 5855577, 5789784, 5658198, 5592405, 5526612, 5460819, 5395026, 5329233, 5263440, 5197647, 5131854, 5066061, 5000268, 4934475, 4868682, 4802889, 4737096, 4671303, 4605510, 4605510, 4539717, 4473924, 4408131, 4342338, 4342338, 4276545, 4210752, 4210752, 4144959, 4079166, 4013373, 4013373, 3947580, 3881787, 3881787, 3815994, 3750201, 3750201, 3684408, 3684408, 3618615, 3552822, 3552822, 3487029, 3487029, 3421236, 3421236, 3355443, 3289650, 3289650, 3223857, 3223857, 3158064, 3158064, 3092271, 3092271, 3026478, 3026478, 2960685, 2960685, 2894892, 2894892, 2829099, 2829099, 2763306, 2763306, 2763306, 2697513, 2697513, 2631720, 2631720, 2565927, 2565927, 2500134, 2500134, 2500134, 2434341, 2434341, 2368548, 2368548, 2368548, 2302755, 2302755, 2236962, 2236962, 2236962, 2171169, 2171169, 2171169, 2105376, 2105376, 2105376, 2039583, 2039583, 1973790, 1973790, 1973790, 1907997, 1907997, 1907997, 1842204, 1842204, 1842204, 1776411, 1776411, 1776411, 1710618, 1710618, 1710618, 1644825, 1644825, 1644825, 1579032, 1579032, 1579032, 1579032, 1513239, 1513239, 1513239, 1447446, 1447446, 1447446, 1381653, 1381653, 1381653, 1381653, 1315860, 1315860, 1315860, 1315860, 1250067, 1250067, 1250067, 1184274, 1184274, 1184274, 1184274, 1118481, 1118481, 1118481, 1118481, 1052688, 1052688, 1052688, 1052688, 986895, 986895, 986895, 921102, 921102, 921102, 921102, 921102, 855309, 855309, 855309, 855309, 789516, 789516, 789516, 789516, 723723, 723723, 723723, 723723, 657930, 657930, 657930, 657930, 657930, 592137, 592137, 592137, 592137, 526344, 526344, 526344, 526344, 526344, 460551, 460551, 460551, 460551, 460551, 394758, 394758, 394758, 394758, 328965, 328965, 328965, 328965, 328965, 263172, 263172, 263172, 263172, 263172, 197379, 197379, 197379, 197379, 197379, 131586, 131586, 131586, 131586, 131586, 131586, 65793, 65793, 65793, 65793, 65793, 0, 0, 0, 0, 0, 0] ("256 log down") u32[] [2155776, 2155776, 2155776, 2155776, 2155776, 2155776, 2155776, 2155776, 127491, 127491, 127491, 127491, 127491, 127491, 127491, 127491, 522752, 522752, 522752, 522752, 522752, 522752, 522752, 522752, 64018, 64018, 64018, 64018, 64018, 64018, 64018, 64018, 63778, 63778, 63778, 63778, 63778, 63778, 63778, 63778, 63790, 63790, 63790, 63790, 63790, 63790, 63790, 63790, 63797, 63797, 63797, 63797, 63797, 63797, 63797, 63797, 63807, 63807, 63807, 63807, 63807, 63807, 63807, 63807, 64068, 64068, 64068, 64068, 64068, 64068, 64068, 64068, 63828, 63828, 63828, 63828, 63828, 63828, 63828, 63828, 63833, 63833, 63833, 63833, 63833, 63833, 63833, 63833, 63836, 63836, 63836, 63836, 63836, 63836, 63836, 63836, 63836, 63836, 63836, 63836, 63836, 63836, 63836, 63836, 61790, 61790, 61790, 61790, 61790, 61790, 61790, 61790, 58464, 58464, 58464, 58464, 58464, 58464, 58464, 58464, 55387, 55387, 55387, 55387, 55387, 55387, 55387, 55387, 51286, 51286, 51286, 51286, 51286, 51286, 51286, 51286, 47440, 47440, 47440, 47440, 47440, 47440, 47440, 47440, 40284, 40284, 40284, 40284, 40284, 40284, 40284, 40284, 34154, 34154, 34154, 34154, 34154, 34154, 34154, 34154, 28540, 28540, 28540, 28540, 28540, 28540, 28540, 28540, 20113, 20113, 20113, 20113, 20113, 20113, 20113, 20113, 12193, 12193, 12193, 12193, 12193, 12193, 12193, 12193, 12714, 12714, 12714, 12714, 12714, 12714, 12714, 12714, 7351, 7351, 7351, 7351, 7351, 7351, 7351, 7351, 4800, 4800, 4800, 4800, 4800, 4800, 4800, 4800, 195, 195, 195, 195, 195, 195, 195, 195, 189, 189, 189, 189, 189, 189, 189, 189, 183, 183, 183, 183, 183, 183, 183, 183, 175, 175, 175, 175, 175, 175, 175, 175, 164, 164, 164, 164, 164, 164, 164, 164, 155, 155, 155, 155, 155, 155, 155, 155] ("32 ice") u32[] [0, 0, 2, 4, 6, 8, 10, 12, 14, 16, 18, 20, 22, 24, 26, 28, 30, 32, 34, 36, 38, 40, 42, 44, 46, 48, 50, 52, 54, 56, 58, 60, 62, 64, 66, 68, 70, 72, 74, 76, 78, 80, 82, 84, 86, 88, 90, 92, 94, 96, 98, 100, 102, 104, 106, 108, 110, 112, 114, 116, 118, 120, 122, 124, 126, 128, 130, 132, 134, 136, 138, 140, 142, 144, 146, 148, 150, 152, 154, 156, 158, 160, 162, 164, 166, 168, 170, 172, 174, 176, 178, 180, 182, 184, 186, 188, 190, 192, 194, 196, 198, 200, 202, 204, 206, 208, 210, 212, 214, 216, 218, 220, 222, 224, 226, 228, 230, 232, 234, 236, 238, 240, 242, 244, 246, 248, 250, 252, 255, 131839, 263423, 395007, 526591, 658175, 789759, 921343, 1052927, 1184511, 1316095, 1447679, 1579263, 1710847, 1842431, 1974015, 2105599, 2237183, 2368767, 2500351, 2631935, 2763519, 2895103, 3026687, 3158271, 3289855, 3421439, 3553023, 3684607, 3816191, 3947775, 4079359, 4210943, 4342527, 4474111, 4605695, 4737279, 4868863, 5000447, 5132031, 5263615, 5395199, 5526783, 5658367, 5789951, 5921535, 6053119, 6184703, 6316287, 6447871, 6579455, 6711039, 6842623, 6974207, 7105791, 7237375, 7368959, 7500543, 7632127, 7763711, 7895295, 8026879, 8158463, 8290047, 8421631, 8553215, 8684799, 8816383, 8947967, 9079551, 9211135, 9342719, 9474303, 9605887, 9737471, 9869055, 10000639, 10132223, 10263807, 10395391, 10526975, 10658559, 10790143, 10921727, 11053311, 11184895, 11316479, 11448063, 11579647, 11711231, 11842815, 11974399, 12105983, 12237567, 12369151, 12500735, 12632319, 12763903, 12895487, 13027071, 13158655, 13290239, 13421823, 13553407, 13684991, 13816575, 13948159, 14079743, 14211327, 14342911, 14474495, 14606079, 14737663, 14869247, 15000831, 15132415, 15263999, 15395583, 15527167, 15658751, 15790335, 15921919, 16053503, 16185087, 16316671, 16448255, 16579839, 16777215] ("original")] -> w81
      frame .."fire" {
      }
      frame "rainbow" {
      }
      frame "grey" {
      }
      frame "inverse grey" {
      }
      frame "ice" {
      }
      frame "original" {
      }
    }
    n89 = Transpose 2D Array(2D array=w90) -> (transposed array=w89:cdb[][])
    n90 = Absolute Value(x=w89) -> (abs(x)=w92:dbl[][])
    n91 = Logarithm Base 10(1:w92) -> (0:w93:dbl[][])
    n92 = Multiply(x=w93, y=i8 20 ("t")) -> (x*y=w95:dbl[][])
    n93 = Array Max & Min(array=w95) -> (max value=w96:dbl)  [unwired: 3 out]
    n94 = Subtract(x=w95, y=w96) -> (x-y=→"ISAR":dbl[][])
    n95 = property on="ISAR" class="IntGraph (strict)"("XScale.Multiplier"=w83, "Color Table"=w81, "ZScale.Maximum"="ISAR intensify: Maximum", "ZScale.Minimum"="ISAR intensify:Minimum", "XScale.Maximum"="range", "YScale.Multiplier"=w75, "YScale.Offset"=w74) -> ()  [unwired: 2 in, 2 out]
  }
  n96 = call <vilib>:"Sound Input Clear.vi"("error in (no error)"=w50, "task ID"=w51) -> ()  [unwired: 9 in, 1 out]
